vi "open TXT file.vi"() -> ()   [LabVIEW 2018, in "Application.lvlib"]
uses:
  Libraries/Application/Application.lvlib
panel:
  out "Array":string[](array[string])
  out "text":string
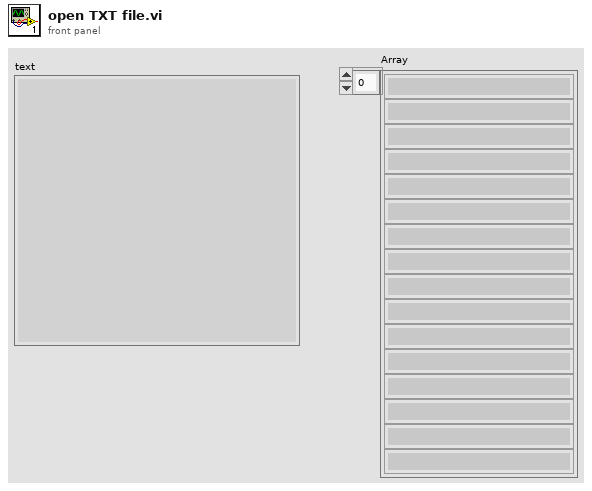
[diagram p1: front panel]
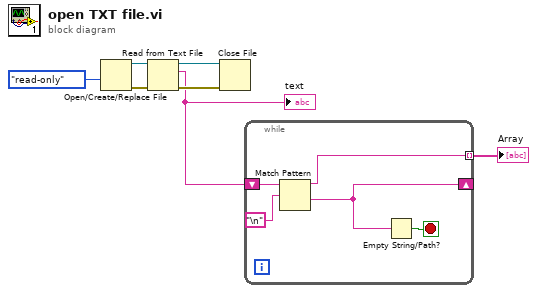
[diagram p0: block diagram]
diagram:
  n1 = Open/Create/Replace File(access (0:read/write)=enum16{"read/write", "read-only", "write-only"}."read-only") -> (refnum out=w6:refnum<file>, error out=w5:errorcluster)  [unwired: 5 in, 1 out]
  n2 = Read from Text File(file (use dialog)=w6, error in=w5) -> (refnum out=w3:refnum<file>, text=w2:string, error out=w4:errorcluster)  [unwired: 2 in, 1 out]
  "text" <- w2
  n3 = Close File(refnum=w3, error in=w4) -> ()  [unwired: 2 out]
  n4 = while {
    shift-right: [w9] -> _
    shift-left: w2 -> [w12]
    tunnel: [w10] -> w1 mode=indexing
    stop <- w8 stop-if-true
    n5 = Match Pattern(string=w12, regular expression="\n") -> (before substring=w10:string, after substring=w9:string)  [unwired: 1 in, 2 out]
    n6 = Empty String/Path?(string/path=w9) -> (empty?=w8:bool)
  }
  "Array" <- w1
